vi "GetTaskList.vi"(8 "error in (no error)":errorcluster, 11 "OrderedList in":refnum<class "TaskList.lvclass">) -> (0 "error out":errorcluster, 2 "TaskList":refnum<class "Collection.lvclass">, 3 "OrderedList out":refnum<class "TaskList.lvclass">)   [LabVIEW 2021, in "LvMarkdown.lvlib" / "TaskList.lvclass"]
uses:
  TaskList.lvclass
  TaskList.lvclass/TaskList.ctl
  Collection/Collection.lvclass
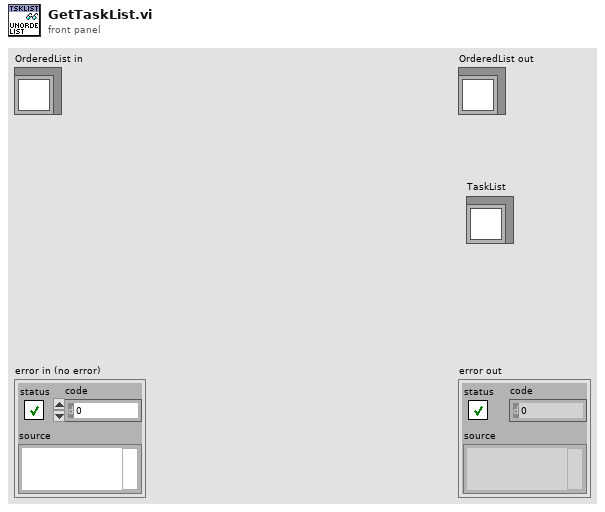
[diagram p1: front panel]
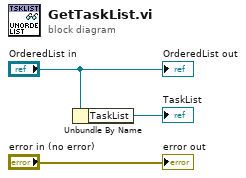
[diagram p0: block diagram]
diagram:
  n1 = Unbundle By Name("OrderedList in") -> ("TaskList"=→"TaskList":refnum<class "Collection.lvclass">)
  "error out" <- "error in (no error)"
  "OrderedList out" <- "OrderedList in"
